vi "(範例)Heat Equation.vi"() -> ()   [LabVIEW 2015]
doc: "This VI simulates the flow of heat across a thin plate from a single point source. The VI solves a well-known elliptic partial differential equation. It demonstrates using MathScript user-defined functions, the 3D scene graph, and mouse interaction with graph cursors."
uses:
  <vilib>/Utility/miscctls.llb/LVPointDoubleTypeDef.ctl
  <vilib>/imath/engines/lvmath2/RunTimeEngine/BuiltInFunctions/ones/NIMS_M=ones(I32,I32).vi
  <vilib>/imathl/engines/lvmath/Functions/Error Handling/Create Error.vi
  <vilib>/imath/engines/lvmath2/RunTimeEngine/NodeEndStatement/NIMS_NodeEndStatement_Output.vi
  <instcachedir>/0/NIMS_NodeEndStatement_Output_53EC0D466D134D7ABD903AC30B43404B.lvgen/NIMS_NodeEndStatement_Output_53EC0D466D134D7ABD903AC30B43404B_002.vi
  <vilib>/imath/engines/lvmath2/RunTimeEngine/ErrorHandling/NIMS_Finalize Error.vi
  Documents/LabVIEW Data/MathScriptVIs/MCStatic_35235434532_9935a2a1c1bf4c8750faca4750d64f77.vi
  <instcachedir>/0/MCStatic_35235434532_9935a2a1c1bf4c8750faca4750d64f77_6041AAA11E25415CADF6CCA159F2CE62.lvgen/MCStatic_35235434532_9935a2a1c1bf4c8750faca4750d64f77_6041AAA11E25415CADF6CCA159F2CE62_000.vi
  <vilib>/imath/engines/lvmath2/RunTimeEngine/ArithmeticOperatorToken/NIMS_ArithmeticOperator_plus.vi
  <instcachedir>/0/NIMS_ArithmeticOperator_plus_A4F2756F5ADB4A0090E0DBD7C10701C8.lvgen/NIMS_ArithmeticOperator_plus_A4F2756F5ADB4A0090E0DBD7C10701C8_003.vi
  <vilib>/imath/engines/lvmath2/RunTimeEngine/ErrorHandling/NIMS_Create Error From Enums.vi
  <vilib>/imath/engines/lvmath2/RunTimeEngine/RangeToken/NIMS_Range.vi
  <instcachedir>/0/NIMS_Range_D919CC09935940E88F755EC1C6F49AC1.lvgen/NIMS_Range_D919CC09935940E88F755EC1C6F49AC1_000.vi
  <vilib>/imath/engines/lvmath2/RunTimeEngine/BuiltInFunctions/meshgrid2d/NIMS_meshgrid2d(V,V).vi
  <instcachedir>/0/NIMS_meshgrid2d(V,V)_3733343E1C554A708015CFB0432C6A59.lvgen/NIMS_meshgrid2d(V,V)_3733343E1C554A708015CFB0432C6A59_000.vi
  <vilib>/imath/engines/lvmath2/RunTimeEngine/VariableToken/Support/NIMS_Vector Boolean Index to I32 Index.vi
  <vilib>/imath/engines/lvmath2/RunTimeEngine/IndexReplace/NIMS V(V)=S.vi
  <instcachedir>/0/NIMS V(V)=S_58A4AA812C6A4554ABBAA1C4D453069D.lvgen/NIMS V(V)=S_58A4AA812C6A4554ABBAA1C4D453069D_000.vi
  <vilib>/imath/engines/lvmath2/RunTimeSupport/NIMS_Error if Not Equal.vi
  <instcachedir>/0/NIMS_Error if Not Equal_7F0D61CE56BF44979916ECA34C78675F.lvgen/NIMS_Error if Not Equal_7F0D61CE56BF44979916ECA34C78675F_001.vi
  <vilib>/imath/engines/lvmath2/RunTimeEngine/IndexRead/NIMS M(V,V).vi
  <instcachedir>/0/NIMS M(V,V)_DD7FAD36288F49D588C120E7830B6EC1.lvgen/NIMS M(V,V)_DD7FAD36288F49D588C120E7830B6EC1_004.vi
  <vilib>/imath/engines/lvmath2/RunTimeEngine/VariableToken/Support/NIMS_Matrix Boolean Index to I32 Index.vi
  <vilib>/imath/engines/lvmath2/RunTimeEngine/IndexReplace/NIMS M(V)=S.vi
  <instcachedir>/0/NIMS M(V)=S_3C8AD9E2E66646CD8081E8D7BAB353DF.lvgen/NIMS M(V)=S_3C8AD9E2E66646CD8081E8D7BAB353DF_000.vi
  <vilib>/imath/engines/lvmath2/RunTimeEngine/IndexReplace/NIMS M(V,V)=M.vi
  <instcachedir>/0/NIMS M(V,V)=M_9544CAF2993349C09F69167D2BA0CD41.lvgen/NIMS M(V,V)=M_9544CAF2993349C09F69167D2BA0CD41_003.vi
  <vilib>/imath/engines/lvmath2/RunTimeEngine/BuiltInFunctions/mean/NIMS_RRow=mean(RM,I32).vi
  <vilib>/imath/engines/lvmath2/RunTimeEngine/BuiltInFunctions/mean/NIMS_RS=mean(RV,I32).vi
  <instcachedir>/0/NIMS_NodeEndStatement_Output_53EC0D466D134D7ABD903AC30B43404B.lvgen/NIMS_NodeEndStatement_Output_53EC0D466D134D7ABD903AC30B43404B_001.vi
  Program Files (x86)/National Instruments/LabVIEW 2015/examples/MathScript/MathScript - Heat Equation/rotatecolumns.m
panel:
  out "Average Temperature":dbl(slide) scale=0.0..100.0
  in  "Point Size":i32(knob)=4 min=0 max=10 step=2 scale=0.0..10.0
  in  "Point Temperature":dbl(slide)=100.0 scale=10.0..100.0
  out "Temperature Field":dbl[][](graph)
  in  "Stop":bool
  in  "Initial Background Temperature":dbl=10.0
  # "Overview: Demonstrates user-defined functions with the MathScript Node, and mouse interaction with graph cursors.\nRequirements: LabVIEW MathScript RT Module\nInstructions:\n1. Run the VI. \n2. Drag the cursor on the Temperature Field graph to move the heat source. \n3. Change the Simulation Parameters to modify the heat source properties.\n4. Click Stop to stop the VI."
  # "Simulation Parameters"
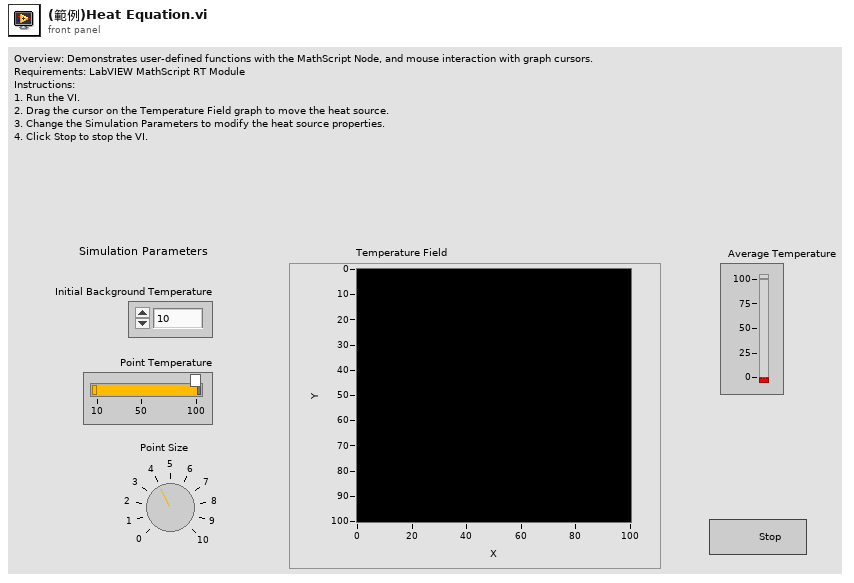
[diagram p1: front panel]
types:
  T1 = typedef "LVPointDoubleTypeDef.ctl" = cluster{"X":dbl, "Y":dbl}
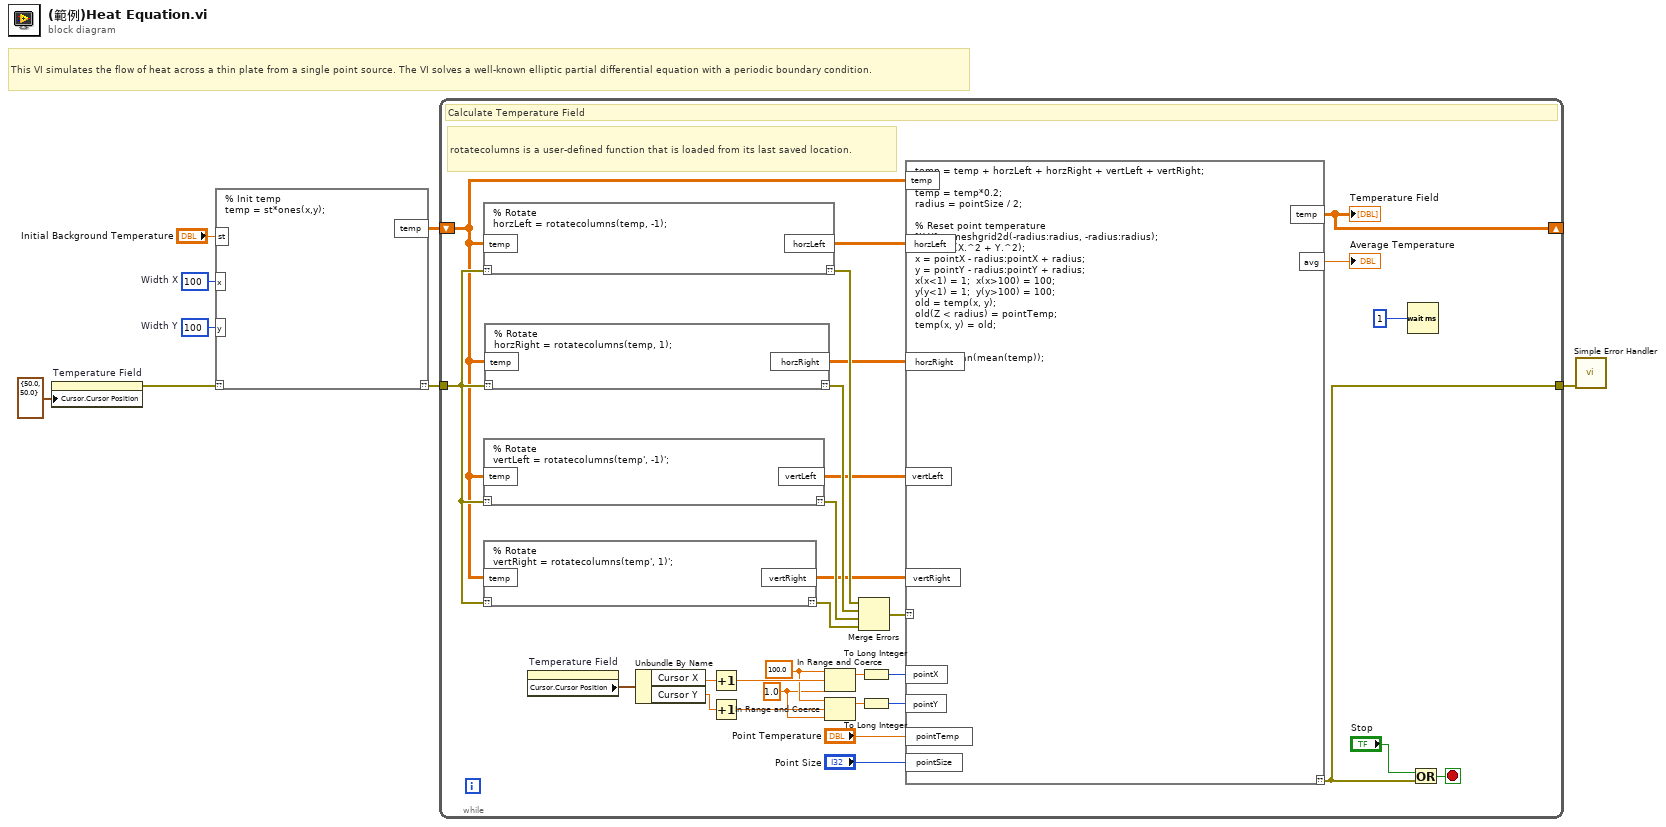
[diagram p0: block diagram]
diagram:
  w5 = 100  # Width Y
  w4 = 100  # Width X
  # "This VI simulates the flow of heat across a thin plate from a single point source. The VI solves a well-known elliptic partial differential equation with a periodic boundary condition."
  n1 = property on="Temperature Field" class="IntGraph (strict)"("Cursor.Cursor Position"=T1 {"X"=50.0, "Y"=50.0}) -> (error out=w2:errorcluster)  [unwired: 2 in, 1 out]
  n2 = mathscript code="% Init temp\ntemp = st*ones(x,y);"("??"=w2, "st"="Initial Background Temperature", "x"=w4, "y"=w5) -> ("??"=w7:errorcluster, "temp"=w6:dbl[][])
  n3 = while {
    shift-right: [w10] -> _
    shift-left: w6 -> [w20]
    tunnel: w7 -> [w26]
    tunnel: [w14] -> w1
    stop <- w38 stop-if-true
    w12 = 100.0 ("Width X")
    w11 = 1.0 ("lower limit")
    # "rotatecolumns is a user-defined function that is loaded from its last saved location."
    # "Calculate Temperature Field"
    n4 = mathscript code="% Rotate\nhorzLeft = rotatecolumns(temp, -1);"("??"=w26, "temp"=w20) -> ("??"=w25:errorcluster, "horzLeft"=w19:dbl[][])
    n5 = mathscript code="% Rotate\nvertLeft = rotatecolumns(temp', -1)';"("??"=w26, "temp"=w20) -> ("??"=w23:errorcluster, "vertLeft"=w17:dbl[][])
    n6 = mathscript code="% Rotate\nvertRight = rotatecolumns(temp', 1)';"("??"=w26, "temp"=w20) -> ("??"=w22:errorcluster, "vertRight"=w16:dbl[][])
    n7 = mathscript code="% Rotate\nhorzRight = rotatecolumns(temp, 1);"("??"=w26, "temp"=w20) -> ("??"=w24:errorcluster, "horzRight"=w18:dbl[][])
    n8 = property on="Temperature Field" class="IntGraph (strict)"() -> ("Cursor.Cursor Position"=w31:T1)  [unwired: 2 in, 2 out]
    n9 = Unbundle By Name(w31) -> ("Cursor X"=w30:dbl, "Cursor Y"=w21:dbl)
    n10 = Increment(x=w30) -> (x+1=w28:dbl)
    n11 = Increment(x=w21) -> (x+1=w27:dbl)
    n12 = In Range and Coerce(upper limit=w12, x=w28, lower limit=w11) -> (coerced(x)=w34:dbl)  [unwired: 1 out]
    n13 = In Range and Coerce(upper limit=w12, x=w27, lower limit=w11) -> (coerced(x)=w33:dbl)  [unwired: 1 out]
    n14 = Merge Errors(w25, w24, w23, w22) -> (w13:errorcluster)
    n15 = To Long Integer(number=w34) -> (32bit integer=w36:i32)
    n16 = To Long Integer(number=w33) -> (32bit integer=w35:i32)
    n17 = mathscript code="temp = temp + horzLeft + horzRight + vertLeft + vertRight;\n\ntemp = temp*0.2;\nradius = pointSize / 2;\n\n% Reset point temperature\n[X Y] = meshgrid2d(-radius:radius, -radius:radius);\nZ = sqrt(X.^2 + Y.^2);\nx = pointX - radius:pointX + radius;\ny = pointY - radius:pointY + radius;\nx(x<1) = 1;  x(x>100) = 100;\ny(y<1) = 1;  y(y>100) = 100;\nold = temp(x, y);\nold(Z < radius) = pointTemp;\ntemp(x, y) = old; \n\n\navg = mean(mean(temp));"("??"=w13, "pointX"=w36, "pointY"=w35, "pointTemp"="Point Temperature", "pointSize"="Point Size", "temp"=w20, "horzLeft"=w19, "horzRight"=w18, "vertLeft"=w17, "vertRight"=w16) -> ("??"=w14:errorcluster, "temp"=w10:dbl[][], "avg"=→"Average Temperature":dbl)
    "Temperature Field" <- w10
    n18 = Wait (ms)(milliseconds to wait=u32 1 ("millisecond multiple")) -> ()  [unwired: 1 out]
    n19 = Or(x="Stop", y=w14) -> (x .or. y?=w38:bool)
  }
  n20 = call <vilib>:"Simple Error Handler.vi"("error in (no error)"=w1) -> ()  [unwired: 4 in, 5 out]
